vi "GetJSONData.vi"(0 "reference in":refnum<class "BooleanControl.lvclass">, 2 "VI Reference":refnum<vi>, 5 "error in (no error)":errorcluster) -> (14 "reference out":refnum<class "BooleanControl.lvclass">, 15 "JSON string":string, 19 "error out":errorcluster)   [LabVIEW 2014, in "BooleanControl.lvclass"]
uses:
  BooleanControl.lvclass
  Control_class/Control.lvclass
  Object_class/Object.lvclass
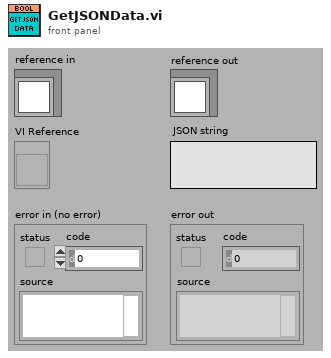
[diagram p1: front panel]
types:
  T1 = typedef "Object.lvclass/Attributes.ctl" = cluster{"UID":i32, "Type":string, "Coordinates":T2}
  T2 = typedef "Object.lvclass/Coordinates.ctl" = cluster{"Left":i32, "Top":i32, "Height":u32, "Width":u32}
  T3 = typedef "Control.lvclass/Attributes.ctl" = cluster{"Description":string, "Indicator":bool, "Default Value":variant, "Control Index":i32, "Label":refnum<class "Text.lvclass">, "Caption":refnum<class "Text.lvclass">, "Use Picture":bool, "Image 1":T4, "Image 2":T4}
  T4 = typedef "imagedata.ctl" = cluster{"image type":i32, "image depth":i32, "image":u8[], "mask":u8[], "colors":u32[], "Rectangle":cluster{"left":i16, "top":i16, "right":i16, "bottom":i16}}
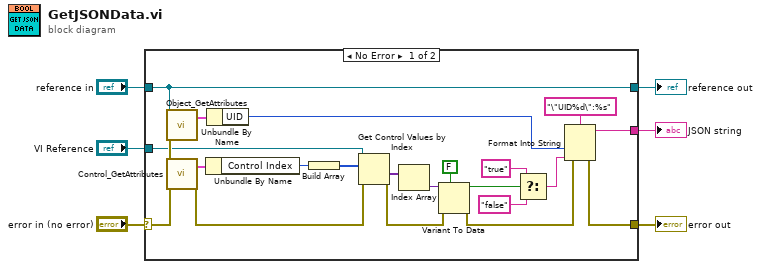
[diagram p0: block diagram]
diagram:
  n1 = case shown="No Error" "error in (no error)" {
    selector: "error in (no error)" -> [w23 w29]
    tunnel: [w24 w29] -> w5
    tunnel: [w9 w28] -> w3
    tunnel: "reference in" -> [w9 w28]
    tunnel: "VI Reference" -> [w17 _]
    tunnel: [w14 _] -> w1
    frame No Error {
      n2 = call "Object_GetAttributes.vi"("reference in"=w9, "error in (no error)"=w23) -> ("Data"=w8:T1)  [unwired: 14 in, 3 out]
      n3 = call "Control_GetAttributes.vi"("reference in"=w9, "error in (no error)"=w23) -> ("Data"=w22:T3, "error out"=w25:errorcluster)  [unwired: 14 in, 2 out]
      n4 = Unbundle By Name(w22) -> ("Control Index"=w21:i32)
      n5 = Unbundle By Name(w8) -> ("UID"=w7:i32)
      n6 = Build Array(w21) -> (w20:i32[])
      n7 = Get Control Values by Index(0:w17, 1:w20, 3:w25) -> (10:w18:variant[], 11:w27:errorcluster)
      n8 = Index Array(array=w18) -> (element=w16:variant)  [unwired: 1 in]
      n9 = Variant To Data(error in=w27, type=FALSE, Variant=w16) -> (data=w13:bool, error out=w26:errorcluster)
      n10 = Select(t="true", s=w13, f="false") -> (s? t:f=w10:string)
      n11 = Format Into String(format string="\"UID%d\":%s", error in=w26, w7, w10) -> (resulting string=w14:string, error out=w24:errorcluster)  [unwired: 1 in]
    }
    frame Error {
    }
  }
  "error out" <- w5
  "reference out" <- w3
  "JSON string" <- w1
